vi "Stop AI.vi"(0 "reference in":refnum<class "AI.lvclass">, 5 "error in (no error)":errorcluster) -> (14 "reference out":refnum<class "AI.lvclass">, 19 "error out":errorcluster)   [LabVIEW 2017, in "AI.lvclass"]
uses:
  AI.lvclass
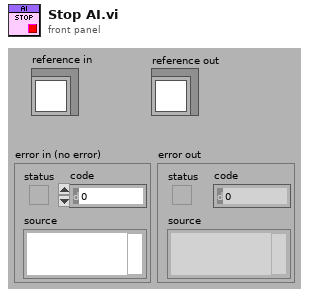
[diagram p1: front panel]
types:
  T1 = typedef "AI.lvclass/ObjectAttributes.ctl" = cluster{"AI Task":refnum<k21>, "AI On/Off Status":bool, "AI Sampling Rate (Samples/Seconds)":u32, "Number of AI Samples Per Channel":i32, "AI Voltage Range":u8, "AI Readings":dbl[][], "Number of AI Modules":i32, "Number of Total AI Channels":i32, "AI Module Names (NI-Max Name)":string[], "Number of Channels Per AI  Module":i32[], "AI VI Reference":refnum<vi>}
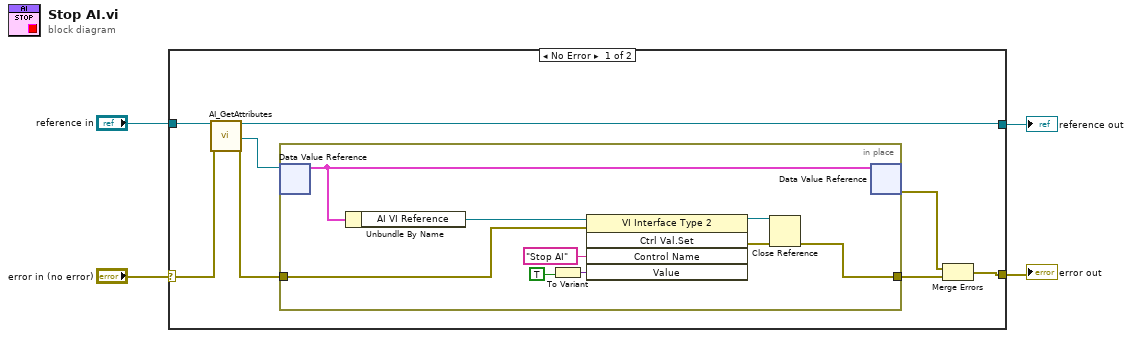
[diagram p0: block diagram]
diagram:
  n1 = case shown="No Error" "error in (no error)" {
    selector: "error in (no error)" -> [w11 w23]
    tunnel: [w8 w23] -> w3
    tunnel: [w9 w22] -> w1
    tunnel: "reference in" -> [w12 w22]
    frame No Error {
      n2 = call "AI_GetAttributes.vi"("reference in"=w12, "error in (no error)"=w11) -> ("reference out"=w9:refnum<class "AI.lvclass">, "DataRef"=w7:refnum<data-value>, "error out"=w6:errorcluster)  [unwired: 14 in, 1 out]
      n3 = in-place {
        in-place-border: w6 -> [w19]
        in-place-border: [w18] -> w5
        n4 = in-place-dvr #1(w7) -> (w13:T1)  [unwired: 1 out]
        n5 = Unbundle By Name(w13) -> ("AI VI Reference"=w21:refnum<vi>)
        n6 = To Variant(anything=TRUE) -> (Variant=w15:variant)
        n7 = invoke class="VI Interface Type 2" method="Ctrl Val.Set"(reference=w21, error in=w19, "Control Name"="Stop AI", "Value"=w15) -> (reference out=w20:refnum<vi>, error out=w17:errorcluster)  [unwired: 1 in, 3 out]
        n8 = Close Reference(reference=w20, error in (no error)=w17) -> (error out=w18:errorcluster)
        n9 = in-place-dvr #1(w13) -> (w10:errorcluster)  [unwired: 1 out]
      }
      n10 = Merge Errors(w10, w5) -> (w8:errorcluster)
    }
    frame Error {
    }
  }
  "error out" <- w3
  "reference out" <- w1
